vi "Set Switch State.vi"(5 "Action":T1(ring)=enum."Connect PulseGen to CH2", 7 "State":bool) -> (15 "error out":errorcluster)   [LabVIEW 2010]
uses:
  <vilib>/DAQmx/write.llb/DAQmx Write (Digital 1D Bool 1Chan 1Samp).vi
  <vilib>/DAQmx/create/channels.llb/DAQmx Create Channel (DO-Digital Output).vi
  <vilib>/daqmx/miscellaneous.llb/DAQmx Fill In Error Info.vi
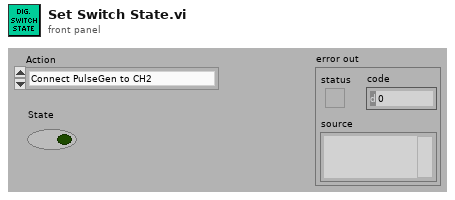
[diagram p1: front panel]
types:
  T1 = enum16{"--Disconnect All--", "Connect PulseGen to CH1", "Connect PulseGen to CH2", "Connect PulseGen to CH3", "Connect PulseGen to CH4", "Connect PulseGen to CH5", "Connect PulseGen to CH6", "Connect PulseGen to CH7", "Connect PulseGen to CH8", "Connect PulseGen to CH9", "Connect PulseGen to CH10", "Connect PulseGen to CH11", "Connect PulseGen to CH12", "Connect PulseGen to CH13", "Connect PulseGen to CH14", "Connect PulseGen to CH15", "Connect PulseGen to CH16", "Connect PulseGen to CH17", "Connect PulseGen to CH18", "Connect PulseGen to CH19", "Connect PulseGen to CH20", "Connect PulseGen to CH21", "Connect PulseGen to CH22", "Connect PulseGen to CH23", "Connect PulseGen to CH24", "Connect PulseGen to CH25", "Set MAG_SW", "Set Dynamic Load", "Set Expansion Trigger", "Trigger Positive Pulse", "Trigger Negative Pulse", "Set MSP Magic Pin", "Set BAT_EN", "Connect MSP_ACLK to CTR", "Connect MSP_MCLK to CTR", "Connect MSP_DIG_TST_OUT to CTR", "Connect STIM_SCK to CTR", "Connect STIM_CLK to CTR", "Connect SMU2 to Magnet", "Magnet Enable", "Cap Short", "Connect Positive Pulse to Pulse Bus", "Connect Negative Pulse to Pulse Bus", "Connect JTAG", "Connect JTAG DVDD Power", "RF Attach", "Connect SMU3 to VBAT", "Connect SMU3 Soft Start", "Connect ARB to Charge Coil", "Connect ARB to Matrix", "Connect CTR to Matrix", "DMM_I Short", "DMM_I 1000 Ohm", "DMM_I 100 Ohm", "DMM_I 10 Ohm", "Connect CH25 to DUT GND"}
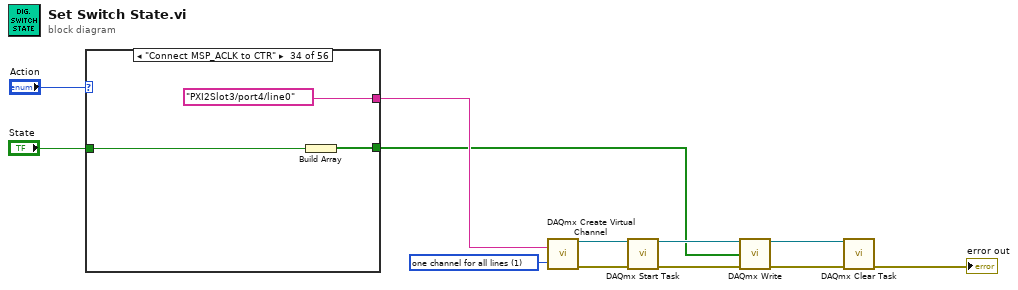
[diagram p0: block diagram]
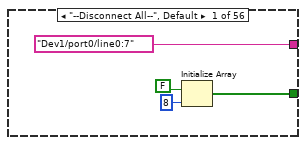
[diagram p2: hidden frame]
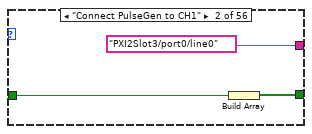
[diagram p3: hidden frame]
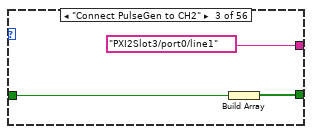
[diagram p4: hidden frame]
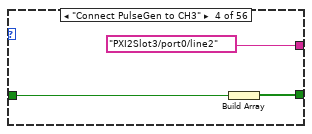
[diagram p5: hidden frame]
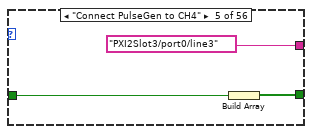
[diagram p6: hidden frame]
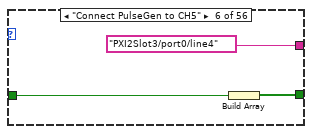
[diagram p7: hidden frame]
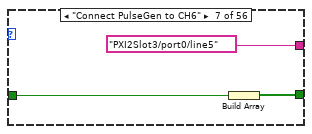
[diagram p8: hidden frame]
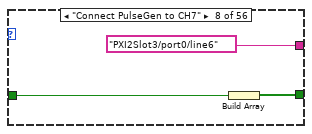
[diagram p9: hidden frame]
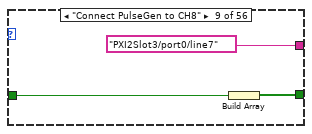
[diagram p10: hidden frame]
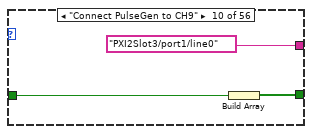
[diagram p11: hidden frame]
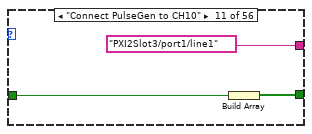
[diagram p12: hidden frame]
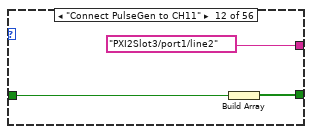
[diagram p13: hidden frame]
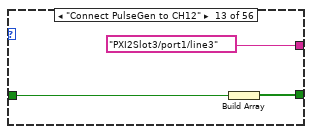
[diagram p14: hidden frame]
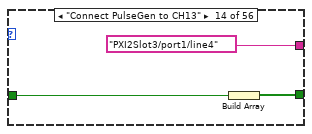
[diagram p15: hidden frame]
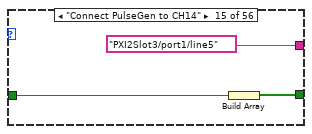
[diagram p16: hidden frame]
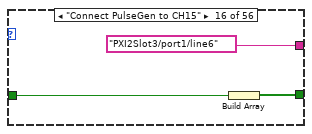
[diagram p17: hidden frame]
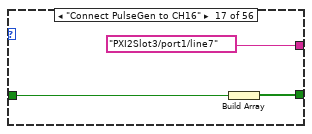
[diagram p18: hidden frame]
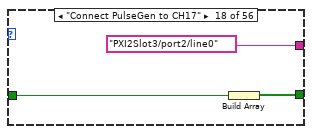
[diagram p19: hidden frame]
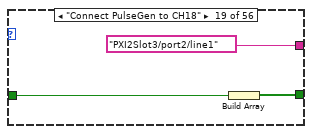
[diagram p20: hidden frame]
diagram:
  w10 = 1 items=["one channel for each line", "one channel for all lines"] ("line grouping")
  n1 = case shown="\"Connect MSP_ACLK to CTR\"" "Action" {
    tunnel: [tag "Dev1/port0/line0:7" ("Lines") tag "PXI2Slot3/port0/line0" ("Lines") tag "PXI2Slot3/port0/line1" ("Lines") tag "PXI2Slot3/port0/line2" ("Lines") tag "PXI2Slot3/port0/line3" ("Lines") tag "PXI2Slot3/port0/line4" ("Lines") tag "PXI2Slot3/port0/line5" ("Lines") tag "PXI2Slot3/port0/line6" ("Lines") tag "PXI2Slot3/port0/line7" ("Lines") tag "PXI2Slot3/port1/line0" ("Lines") tag "PXI2Slot3/port1/line1" ("Lines") tag "PXI2Slot3/port1/line2" ("Lines") tag "PXI2Slot3/port1/line3" ("Lines") tag "PXI2Slot3/port1/line4" ("Lines") tag "PXI2Slot3/port1/line5" ("Lines") tag "PXI2Slot3/port1/line6" ("Lines") tag "PXI2Slot3/port1/line7" ("Lines") tag "PXI2Slot3/port2/line0" ("Lines") tag "PXI2Slot3/port2/line1" ("Lines") tag "PXI2Slot3/port2/line2" ("Lines") tag "PXI2Slot3/port2/line3" ("Lines") tag "PXI2Slot3/port2/line4" ("Lines") tag "PXI2Slot3/port2/line5" ("Lines") tag "PXI2Slot3/port2/line6" ("Lines") tag "PXI2Slot3/port2/line7" ("Lines") tag "PXI2Slot3/port3/line0" ("Lines") tag "PXI2Slot3/port3/line1" ("Lines") tag "PXI2Slot3/port3/line2:3" ("Lines") tag "PXI2Slot3/port3/line3" ("Lines") tag "PXI2Slot3/port3/line3:4" ("Lines") tag "PXI2Slot3/port3/line3:5" ("Lines") tag "PXI2Slot3/port3/line6" ("Lines") tag "PXI2Slot3/port3/line7" ("Lines") tag "PXI2Slot3/port4/line0" ("Lines") tag "PXI2Slot3/port4/line1" ("Lines") tag "PXI2Slot3/port4/line2" ("Lines") tag "PXI2Slot3/port4/line3" ("Lines") tag "PXI2Slot3/port4/line4" ("Lines") tag "PXI2Slot3/port4/line5" ("Lines") tag "PXI2Slot3/port4/line6" ("Lines") tag "PXI2Slot3/port4/line7" ("Lines") tag "PXI2Slot3/port5/line0" ("Lines") tag "PXI2Slot3/port5/line1" ("Lines") tag "PXI2Slot3/port5/line2" ("Lines") tag "PXI2Slot3/port5/line3" ("Lines") tag "PXI2Slot3/port5/line4" ("Lines") tag "PXI2Slot3/port5/line5" ("Lines") tag "PXI2Slot3/port5/line6" ("Lines") tag "PXI2Slot3/port5/line7" ("Lines") tag "PXI2Slot3/port6/line7" ("Lines") tag "PXI2Slot3/port6/line6" ("Lines") tag "PXI2Slot3/port6/line5" ("Lines") tag "PXI2Slot3/port6/line4" ("Lines") tag "PXI2Slot3/port6/line3" ("Lines") tag "PXI2Slot3/port6/line2" ("Lines") tag "PXI2Slot3/port6/line1" ("Lines")] -> w4
    tunnel: [w13 w18 w21 w24 w27 w30 w33 w36 w39 w42 w45 w48 w51 w54 w57 w60 w63 w66 w69 w72 w75 w78 w81 w84 w87 w90 w93 w96 w99 w102 w106 w109 w112 w115 w118 w121 w124 w127 w130 w133 w136 w139 w142 w145 w148 w151 w154 w157 w160 w163 w166 w169 w172 w175 w178 w181] -> w3
    tunnel: "State" -> [_ w17 w20 w23 w26 w29 w32 w35 w38 w41 w44 w47 w50 w53 w56 w59 w62 w65 w68 w71 w74 w77 w80 w83 w86 w89 w92 w95 w98 w101 w105 w108 w111 w114 w117 w120 w123 w126 w129 w132 w135 w138 w141 w144 w147 w150 w153 w156 w159 w162 w165 w168 w171 w174 w177 w180]
    frame "--Disconnect All--", Default {
      n2 = Initialize Array(FALSE, 8 ("dimension size")) -> (w13:bool[])
    }
    frame "Connect PulseGen to CH1" {
      n3 = Build Array(w17) -> (w18:bool[])
    }
    frame "Connect PulseGen to CH2" {
      n4 = Build Array(w20) -> (w21:bool[])
    }
    frame "Connect PulseGen to CH3" {
      n5 = Build Array(w23) -> (w24:bool[])
    }
    frame "Connect PulseGen to CH4" {
      n6 = Build Array(w26) -> (w27:bool[])
    }
    frame "Connect PulseGen to CH5" {
      n7 = Build Array(w29) -> (w30:bool[])
    }
    frame "Connect PulseGen to CH6" {
      n8 = Build Array(w32) -> (w33:bool[])
    }
    frame "Connect PulseGen to CH7" {
      n9 = Build Array(w35) -> (w36:bool[])
    }
    frame "Connect PulseGen to CH8" {
      n10 = Build Array(w38) -> (w39:bool[])
    }
    frame "Connect PulseGen to CH9" {
      n11 = Build Array(w41) -> (w42:bool[])
    }
    frame "Connect PulseGen to CH10" {
      n12 = Build Array(w44) -> (w45:bool[])
    }
    frame "Connect PulseGen to CH11" {
      n13 = Build Array(w47) -> (w48:bool[])
    }
    frame "Connect PulseGen to CH12" {
      n14 = Build Array(w50) -> (w51:bool[])
    }
    frame "Connect PulseGen to CH13" {
      n15 = Build Array(w53) -> (w54:bool[])
    }
    frame "Connect PulseGen to CH14" {
      n16 = Build Array(w56) -> (w57:bool[])
    }
    frame "Connect PulseGen to CH15" {
      n17 = Build Array(w59) -> (w60:bool[])
    }
    frame "Connect PulseGen to CH16" {
      n18 = Build Array(w62) -> (w63:bool[])
    }
    frame "Connect PulseGen to CH17" {
      n19 = Build Array(w65) -> (w66:bool[])
    }
    frame "Connect PulseGen to CH18" {
      n20 = Build Array(w68) -> (w69:bool[])
    }
    frame "Connect PulseGen to CH19" {
      n21 = Build Array(w71) -> (w72:bool[])
    }
    frame "Connect PulseGen to CH20" {
      n22 = Build Array(w74) -> (w75:bool[])
    }
    frame "Connect PulseGen to CH21" {
      n23 = Build Array(w77) -> (w78:bool[])
    }
    frame "Connect PulseGen to CH22" {
      n24 = Build Array(w80) -> (w81:bool[])
    }
    frame "Connect PulseGen to CH23" {
      n25 = Build Array(w83) -> (w84:bool[])
    }
    frame "Connect PulseGen to CH24" {
      n26 = Build Array(w86) -> (w87:bool[])
    }
    frame "Connect PulseGen to CH25" {
      n27 = Build Array(w89) -> (w90:bool[])
    }
    frame "Set MAG_SW" {
      n28 = Build Array(w92) -> (w93:bool[])
    }
    frame "Set Dynamic Load" {
      n29 = Build Array(w95, w95) -> (w96:bool[])
    }
    frame "Set Expansion Trigger" {
      n30 = Build Array(w98) -> (w99:bool[])
    }
    frame "Trigger Positive Pulse" {
      n31 = Build Array(w101, w101) -> (w102:bool[])
    }
    frame "Trigger Negative Pulse" {
      n32 = Build Array(w105, FALSE ("element"), w105) -> (w106:bool[])
    }
    frame "Set MSP Magic Pin" {
      n33 = Build Array(w108) -> (w109:bool[])
    }
    frame "Set BAT_EN" {
      n34 = Build Array(w111) -> (w112:bool[])
    }
    frame "Connect MSP_ACLK to CTR" {
      n35 = Build Array(w114) -> (w115:bool[])
    }
    frame "Connect MSP_MCLK to CTR" {
      n36 = Build Array(w117) -> (w118:bool[])
    }
    frame "Connect MSP_DIG_TST_OUT to CTR" {
      n37 = Build Array(w120) -> (w121:bool[])
    }
    frame "Connect STIM_SCK to CTR" {
      n38 = Build Array(w123) -> (w124:bool[])
    }
    frame "Connect STIM_CLK to CTR" {
      n39 = Build Array(w126) -> (w127:bool[])
    }
    frame "Connect SMU2 to Magnet" {
      n40 = Build Array(w129) -> (w130:bool[])
    }
    frame "Magnet Enable" {
      n41 = Build Array(w132) -> (w133:bool[])
    }
    frame "Cap Short" {
      n42 = Build Array(w135) -> (w136:bool[])
    }
    frame "Connect Positive Pulse to Pulse Bus" {
      n43 = Build Array(w138) -> (w139:bool[])
    }
    frame "Connect Negative Pulse to Pulse Bus" {
      n44 = Build Array(w141) -> (w142:bool[])
    }
    frame "Connect JTAG" {
      n45 = Build Array(w144) -> (w145:bool[])
    }
    frame "Connect JTAG DVDD Power" {
      n46 = Build Array(w147) -> (w148:bool[])
    }
    frame "RF Attach" {
      n47 = Build Array(w150) -> (w151:bool[])
    }
    frame "Connect SMU3 to VBAT" {
      n48 = Build Array(w153) -> (w154:bool[])
    }
    frame "Connect SMU3 Soft Start" {
      n49 = Build Array(w156) -> (w157:bool[])
    }
    frame "Connect ARB to Charge Coil" {
      n50 = Build Array(w159) -> (w160:bool[])
    }
    frame "Connect ARB to Matrix" {
      n51 = Build Array(w162) -> (w163:bool[])
    }
    frame "Connect CTR to Matrix" {
      n52 = Build Array(w165) -> (w166:bool[])
    }
    frame "DMM_I Short" {
      n53 = Build Array(w168) -> (w169:bool[])
    }
    frame "DMM_I 1000 Ohm" {
      n54 = Build Array(w171) -> (w172:bool[])
    }
    frame "DMM_I 100 Ohm" {
      n55 = Build Array(w174) -> (w175:bool[])
    }
    frame "DMM_I 10 Ohm" {
      n56 = Build Array(w177) -> (w178:bool[])
    }
    frame "Connect CH25 to DUT GND" {
      n57 = Build Array(w180) -> (w181:bool[])
    }
  }
  n58 = call-poly <vilib>:"DAQmx Create Virtual Channel.vi"("lines"=w4, "line grouping"=w10) -> ("task out"=w12:refnum<k21>, "error out"=w11:errorcluster)  [unwired: 12 in]
  n59 = call <vilib>:"DAQmx Start Task.vi"("task/channels in"=w12, "error in"=w11) -> ("task out"=w9:refnum<k21>, "error out"=w8:errorcluster)  [unwired: 12 in]
  n60 = call-poly <vilib>:"DAQmx Write.vi"("task/channels in"=w9, "data"=w3, "error in"=w8) -> ("task out"=w7:refnum<k21>, "error out"=w6:errorcluster)  [unwired: 10 in, 1 out]
  n61 = call <vilib>:"DAQmx Clear Task.vi"("task in"=w7, "error in"=w6) -> ("error out"=→"error out":errorcluster)  [unwired: 13 in]
